vi "INI_Dialog display options.vi"(7 "File Action":enum16{"Read", "Write"}(ring), 11 "Display Options":T1) -> (3 "Display Options Out":T1)   [LabVIEW 2023]
uses:
  <userlib>/_OpenG.lib/variantconfig/variantconfig.llb/openg_variant_configuration_file.lvlib
  <vilib>/Utility/config.llb/NI_LVConfig.lvlib
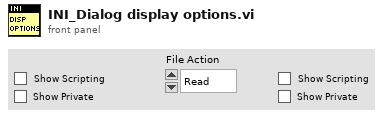
[diagram p1: front panel]
types:
  T1 = cluster{"Show Scripting":bool, "Show Private":bool}
  T2 = typedef "NI_LVConfig.lvlib/Config Data RefNum.ctl" = refnum<k1>
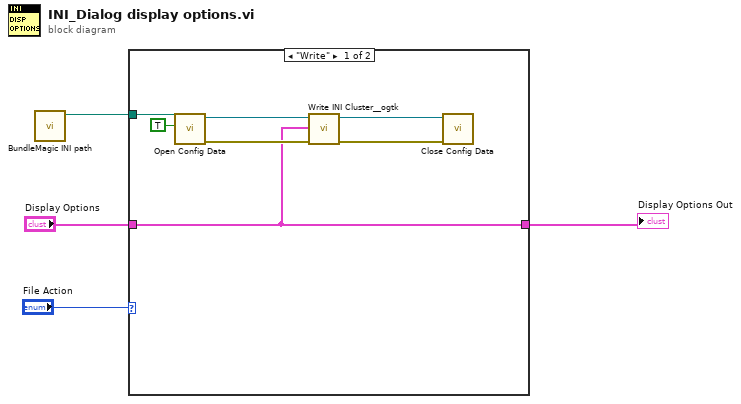
[diagram p0: block diagram]
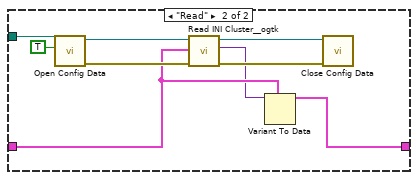
[diagram p2: hidden frame]
diagram:
  n1 = call "BundleMagic INI path.vi"() -> ("appended path"=w1:path)  [unwired: 11 in]
  n2 = case shown="\"Write\"" "File Action" {
    tunnel: w1 -> [w7 w16]
    tunnel: "Display Options" -> [w5 w14]
    tunnel: [w5 w12] -> w2
    frame "Write" {
      n3 = call <vilib>:"Open Config Data.vi"("create file if necessary (T)"=TRUE, "configuration file path"=w7) -> ("error out"=w9:errorcluster, "refnum"=w11:T2)  [unwired: 7 in, 1 out]
      n4 = call <userlib>:"Write INI Cluster__ogtk.vi"("error in (no error)"=w9, "INI Fomatted Cluster"=w5, "refnum"=w11) -> ("error out"=w8:errorcluster, "dup refnum"=w10:T2)  [unwired: 7 in]
      n5 = call <vilib>:"Close Config Data.vi"("error in (no error)"=w8, "refnum"=w10) -> ()  [unwired: 8 in, 2 out]
    }
    frame "Read" {
      n6 = call <vilib>:"Open Config Data.vi"("create file if necessary (T)"=TRUE, "configuration file path"=w16) -> ("error out"=w18:errorcluster, "refnum"=w20:T2)  [unwired: 7 in, 1 out]
      n7 = call <userlib>:"Read INI Cluster__ogtk.vi"("error in (no error)"=w18, "INI Fomatted Cluster Type"=w14, "refnum"=w20) -> ("error out"=w17:errorcluster, "INI Fomatted Cluster"=w13:variant, "dup refnum"=w19:T2)  [unwired: 4 in, 2 out]
      n8 = Variant To Data(type=w14, Variant=w13) -> (data=w12:T1)  [unwired: 1 in, 1 out]
      n9 = call <vilib>:"Close Config Data.vi"("error in (no error)"=w17, "refnum"=w19) -> ()  [unwired: 8 in, 2 out]
    }
  }
  "Display Options Out" <- w2
